vi "SetJogType.vi"(8 "error in (no error)":errorcluster, 10 "JogMode":i16(ring)=1 items=["ContinuousHeld"=1, "SingleStep"=2, "ContinuousUnheld"=3], 11 "ThorlabsLabJack in":refnum<class "ThorlabsLabJack.lvclass">) -> (0 "error out":errorcluster, 3 "ThorlabsLabJack out":refnum<class "ThorlabsLabJack.lvclass">)   [LabVIEW 2018, in "ThorlabsLabJack.lvlib" / "ThorlabsLabJack.lvclass"]
uses:
  ThorlabsLabJack.lvclass
  ThorlabsLabJack.lvclass/ThorlabsLabJack.ctl
  C:/Projects/LabVIEW/In-Progress/Chetan Malpure/Axis/Thorlabs LabJack/Drivers/Thorlabs.MotionControl.IntegratedStepperMotorsCLI.dll
  Drivers/Thorlabs.MotionControl.IntegratedStepperMotorsCLI.dll
  C:/Projects/LabVIEW/In-Progress/Chetan Malpure/Axis/Thorlabs LabJack/Drivers/Thorlabs.MotionControl.GenericMotorCLI.dll
  Drivers/Thorlabs.MotionControl.GenericMotorCLI.dll
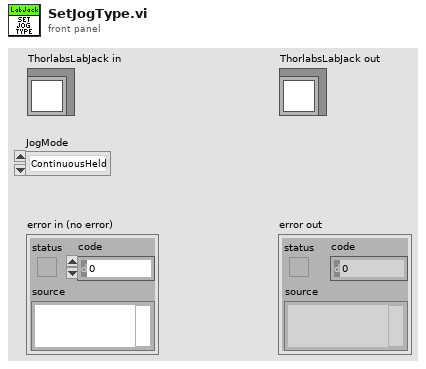
[diagram p1: front panel]
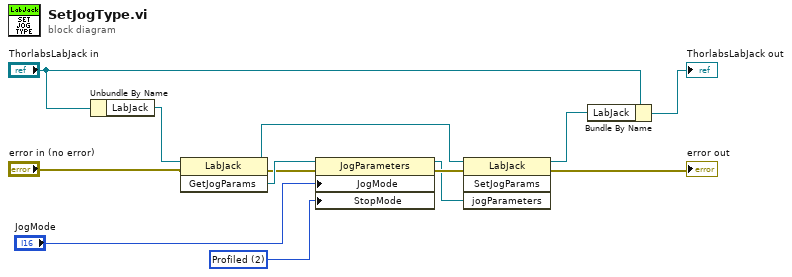
[diagram p0: block diagram]
diagram:
  w6 = i16 2 items=["Immediate"=1, "Profiled"=2] ("StopMode")
  n1 = Unbundle By Name("ThorlabsLabJack in") -> ("LabJack"=w11:refnum<k24>)
  n2 = invoke class="LabJack" method="GetJogParams"(reference=w11, error in="error in (no error)") -> (reference out=w4:refnum<k24>, error out=w8:errorcluster, "GetJogParams"=w9:refnum<k24>)  [unwired: 1 in]
  n3 = property class="JogParameters"(reference=w9, error in=w8, "JogMode"="JogMode", "StopMode"=w6) -> (reference out=w3:refnum<k24>, error out=w5:errorcluster)
  n4 = invoke class="LabJack" method="SetJogParams"(reference=w4, error in=w5, "jogParameters"=w3) -> (reference out=w2:refnum<k24>, error out=→"error out":errorcluster)  [unwired: 1 in, 2 out]
  n5 = Bundle By Name(cluster="ThorlabsLabJack in", "LabJack"=w2) -> (→"ThorlabsLabJack out":refnum<class "ThorlabsLabJack.lvclass">)
